vi "ctet_mux_User Main.vi"() -> ()   [LabVIEW 2019, in "ctet_mux_User Library.lvlib"]
uses:
  ctet_mux_User Library.lvlib
  Servers/ctet_mux/ctet_mux Class/typeDefs/Server State Data.ctl
  Types/ctet_mux.ctl
  Servers/ctet_mux/ctet_mux Class/ctet_mux.lvclass/ctet_mux.ctl
  Servers/ctet_mux/ctet_mux Class/ctet_mux.lvclass
panel:
  in  "Stop":bool
  in  "Server Address":string="0.0.0.0:50051"
  in  "Server Certificate File (.crt)":path
  in  "Server Key File (.key)":path
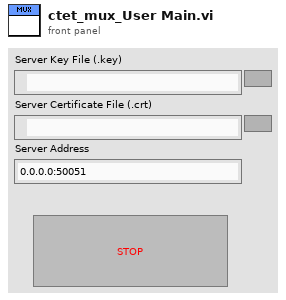
[diagram p1: front panel]
types:
  T1 = typedef "ctet_mux_User Library.lvlib/ctet_mux.ctl" = cluster{"MUXSession":refnum<k15>}
  T2 = typedef "ctet_mux.lvlib/ctet_mux.lvclass/Server State Data.ctl" = cluster{"Data":string}
  T3 = typedef "ctet_mux.lvlib/ctet_mux.lvclass/Server gRPC UEs.ctl" = cluster{"Invoke gRPC UE":refnum<user-event>, "Query gRPC UE":refnum<user-event>, "Register gRPC UE":refnum<user-event>, "OpenMUXSession gRPC UE":refnum<user-event>, "CloseMUXSession gRPC UE":refnum<user-event>, "OpenMUXChannel gRPC UE":refnum<user-event>, "CloseMUXChannel gRPC UE":refnum<user-event>, "OpenMUXRelay gRPC UE":refnum<user-event>, "CloseMUXRelay gRPC UE":refnum<user-event>, "CloseMUXAllRelays gRPC UE":refnum<user-event>, "DisconnectAllMUXChannels gRPC UE":refnum<user-event>, "ResetMUX gRPC UE":refnum<user-event>, "GetMUXStatus gRPC UE":refnum<user-event>, "GetMUXChannelNames gRPC UE":refnum<user-event>, "GetMUXRelayInfo gRPC UE":refnum<user-event>}
  T4 = typedef "ctet_mux.lvlib/gprc-lvsupport.lvlib/grpcId.ctl" = u64
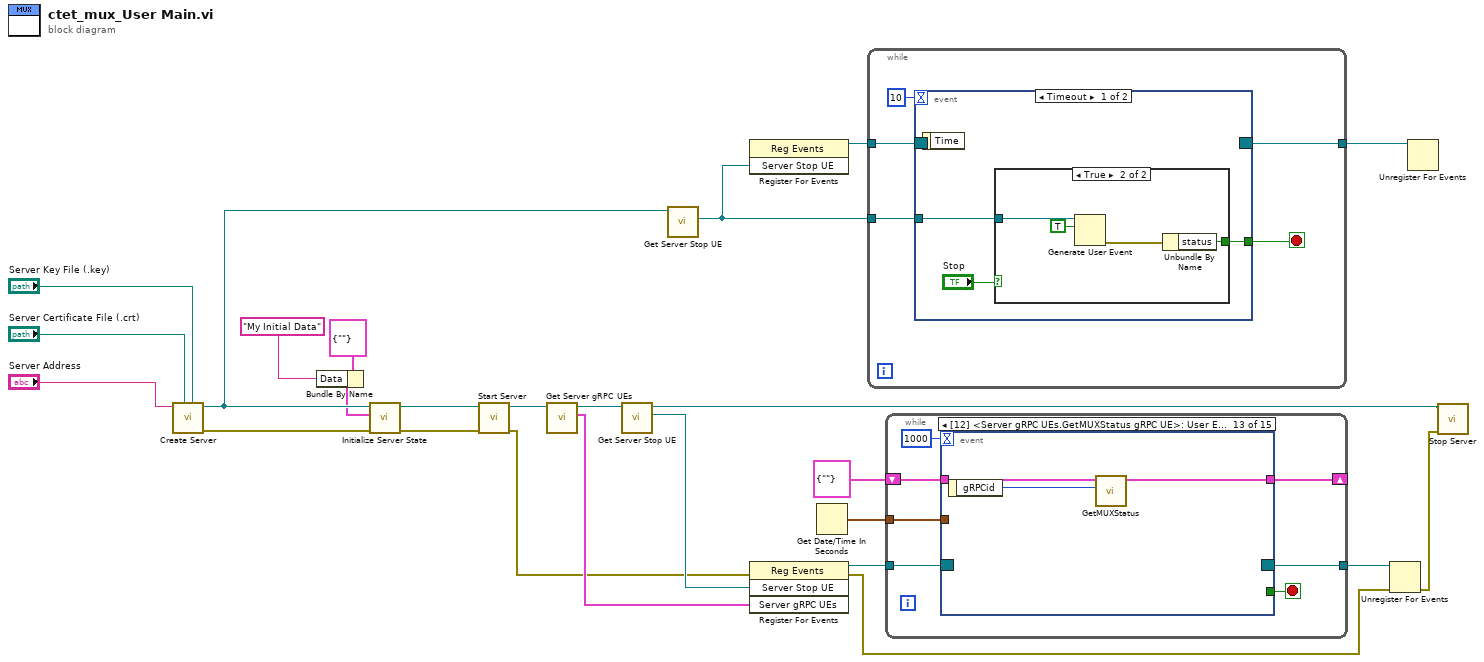
[diagram p0: block diagram]
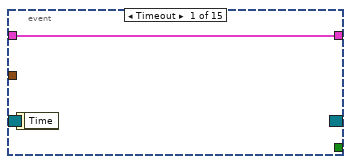
[diagram p2: hidden frame]
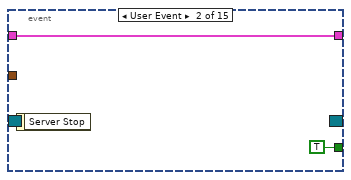
[diagram p3: hidden frame]
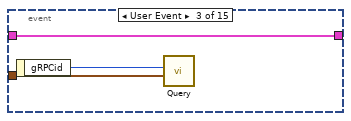
[diagram p4: hidden frame]
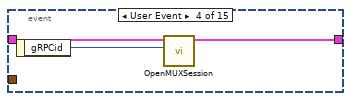
[diagram p5: hidden frame]
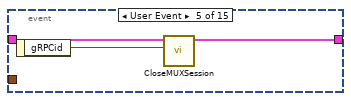
[diagram p6: hidden frame]
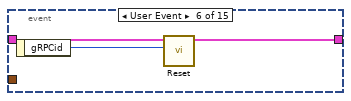
[diagram p7: hidden frame]
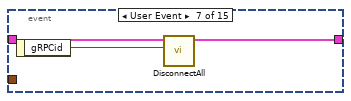
[diagram p8: hidden frame]
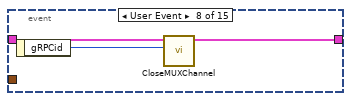
[diagram p9: hidden frame]
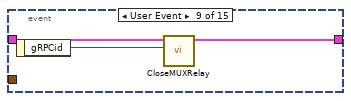
[diagram p10: hidden frame]
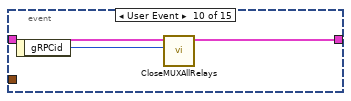
[diagram p11: hidden frame]
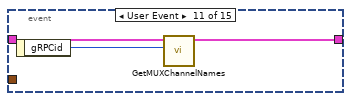
[diagram p12: hidden frame]
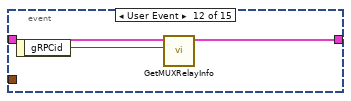
[diagram p13: hidden frame]
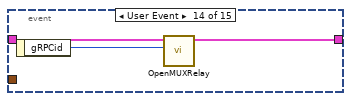
[diagram p14: hidden frame]
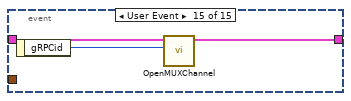
[diagram p15: hidden frame]
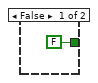
[diagram p16: hidden frame]
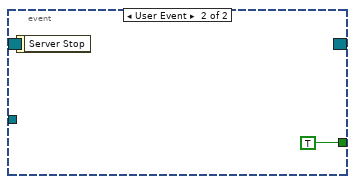
[diagram p17: hidden frame]
diagram:
  n1 = call "Create Server.vi"("Server Key File (.key)"="Server Key File (.key)", "Server Certificate File (.crt)"="Server Certificate File (.crt)", "Server Address"="Server Address") -> ("error out"=w19:errorcluster, "gRPC Server out"=w16:refnum<class "ctet_mux.lvclass">)  [unwired: 7 in]
  n2 = Bundle By Name(cluster=T2 {"Data"=""} ("Initial State"), "Data"="My Initial Data") -> (w14:T2)
  n3 = call "Initialize Server State.vi"("error in (no error)"=w19, "Initial State"=w14, "gRPC Server in"=w16) -> ("error out"=w18:errorcluster, "gRPC Server out"=w17:refnum<class "ctet_mux.lvclass">)  [unwired: 7 in]
  n4 = call "Start Server.vi"("error in (no error)"=w18, "gRPC Server in"=w17) -> ("error out"=w6:errorcluster, "gRPC Server out"=w7:refnum<class "ctet_mux.lvclass">)  [unwired: 8 in]
  n5 = call "Get Server gRPC UEs.vi"("OOP Server in"=w7) -> ("Server gRPC UEs"=w10:T3, "OOP Server out"=w12:refnum<class "ctet_mux.lvclass">)  [unwired: 9 in]
  n6 = call "Get Server Stop UE.vi"("OOP Server in"=w12) -> ("Server Stop UE"=w11:refnum<user-event>, "OOP Server out"=w4:refnum<class "ctet_mux.lvclass">)  [unwired: 9 in]
  n7 = call "Get Server Stop UE.vi"("OOP Server in"=w16) -> ("Server Stop UE"=w20:refnum<user-event>)  [unwired: 9 in, 1 out]
  n8 = register-events(w20) -> (reference out=w22:refnum<event-registration>)  [unwired: 2 in, 1 out]
  n9 = register-events(error in=w6, w11, w10) -> (reference out=w9:refnum<event-registration>, error out=w5:errorcluster)  [unwired: 1 in]
  n10 = Get Date/Time In Seconds() -> (seconds since 1Jan1904=w2:timestamp)
  n11 = while {
    tunnel: w20 -> [w30]
    tunnel: w22 -> [w29]
    tunnel: [w27] -> w21
    stop <- w28 stop-if-true
    n12 = event shown="[0] Timeout" {
      selector: w29 -> [_ _]
      dyn-events: [_ _] -> w27
      timeout: 10 -> [_ _]
      tunnel: w30 -> [w33 _]
      tunnel: [w32 TRUE] -> w28
      event Timeout {
        n13 = event-data() -> ()  [unwired: 1 in, 1 out]
        n14 = case shown="True" "Stop" {
          tunnel: w33 -> [_ w36]
          tunnel: [FALSE ("status") w35] -> w32
          frame False {
          }
          frame True {
            n15 = Generate User Event(user event=w36, event data cluster=TRUE ("event data")) -> (error out=w37:errorcluster)  [unwired: 2 in, 1 out]
            n16 = Unbundle By Name(w37) -> ("status"=w35:bool)
          }
        }
      }
      event User Event {
        n17 = event-data() -> ()  [unwired: 1 in, 1 out]
      }
    }
  }
  n18 = while {
    tunnel: w9 -> [w46]
    tunnel: [w44] -> w8
    tunnel: w2 -> [w42]
    shift-right: [w40] -> _
    shift-left: T1 {"MUXSession"=""} ("ctet_mux in") -> [w41]
    stop <- w45 stop-if-true
    n19 = event "RPC Methods Event Structure" shown="[12] <Server gRPC UEs.GetMUXStatus gRPC UE>: User Event" {
      selector: w46 -> [_ _ _ _ _ _ _ _ _ _ _ _ _ _ _]
      dyn-events: [_ _ _ _ _ _ _ _ _ _ _ _ _ _ _] -> w44
      timeout: 1000 -> [_ _ _ _ _ _ _ _ _ _ _ _ _ _ _]
      tunnel: [_ TRUE _ _ _ _ _ _ _ _ _ _ _ _ _] -> w45
      tunnel: w42 -> [_ _ w51 _ _ _ _ _ _ _ _ _ _ _ _]
      tunnel: w41 -> [w47 w48 w50 w54 w57 w60 w63 w66 w69 w72 w75 w78 w81 w84 w87]
      tunnel: [w47 w48 w50 w53 w56 w59 w62 w65 w68 w71 w74 w77 w80 w83 w86] -> w40
      event Timeout {
        n20 = event-data() -> ()  [unwired: 1 in, 1 out]
      }
      event User Event {
        n21 = event-data() -> ()  [unwired: 1 in, 1 out]
      }
      event User Event {
        n22 = event-data() -> ("gRPCid"=w52:T4)  [unwired: 1 in]
        n23 = call "Query.vi"("current time"=w51, "gRPCid"=w52) -> ()  [unwired: 9 in, 1 out]
      }
      event User Event {
        n24 = event-data() -> ("gRPCid"=w55:T4)  [unwired: 1 in]
        n25 = call "OpenMUXSession.vi"("gRPCid"=w55, "ctet_mux in"=w54) -> ("ctet_mux out"=w53:T1)  [unwired: 8 in, 1 out]
      }
      event User Event {
        n26 = event-data() -> ("gRPCid"=w58:T4)  [unwired: 1 in]
        n27 = call "CloseMUXSession.vi"("gRPCid"=w58, "ctet_mux in"=w57) -> ("ctet_mux out"=w56:T1)  [unwired: 8 in, 1 out]
      }
      event User Event {
        n28 = event-data() -> ("gRPCid"=w61:T4)  [unwired: 1 in]
        n29 = call "Reset.vi"("gRPCid"=w61, "ctet_mux in"=w60) -> ("ctet_mux out"=w59:T1)  [unwired: 8 in, 1 out]
      }
      event User Event {
        n30 = event-data() -> ("gRPCid"=w64:T4)  [unwired: 1 in]
        n31 = call "DisconnectAll.vi"("gRPCid"=w64, "ctet_mux in"=w63) -> ("ctet_mux out"=w62:T1)  [unwired: 8 in, 1 out]
      }
      event User Event {
        n32 = event-data() -> ("gRPCid"=w67:T4)  [unwired: 1 in]
        n33 = call "CloseMUXChannel.vi"("gRPCid"=w67, "ctet_mux in"=w66) -> ("ctet_mux out"=w65:T1)  [unwired: 8 in, 1 out]
      }
      event User Event {
        n34 = event-data() -> ("gRPCid"=w70:T4)  [unwired: 1 in]
        n35 = call "CloseMUXRelay.vi"("gRPCid"=w70, "ctet_mux in"=w69) -> ("ctet_mux out"=w68:T1)  [unwired: 8 in, 1 out]
      }
      event User Event {
        n36 = event-data() -> ("gRPCid"=w73:T4)  [unwired: 1 in]
        n37 = call "CloseMUXAllRelays.vi"("gRPCid"=w73, "ctet_mux in"=w72) -> ("ctet_mux out"=w71:T1)  [unwired: 8 in, 1 out]
      }
      event User Event {
        n38 = event-data() -> ("gRPCid"=w76:T4)  [unwired: 1 in]
        n39 = call "GetMUXChannelNames.vi"("gRPCid"=w76, "ctet_mux in"=w75) -> ("ctet_mux out"=w74:T1)  [unwired: 8 in, 1 out]
      }
      event User Event {
        n40 = event-data() -> ("gRPCid"=w79:T4)  [unwired: 1 in]
        n41 = call "GetMUXRelayInfo.vi"("gRPCid"=w79, "ctet_mux in"=w78) -> ("ctet_mux out"=w77:T1)  [unwired: 8 in, 1 out]
      }
      event User Event {
        n42 = event-data() -> ("gRPCid"=w82:T4)  [unwired: 1 in]
        n43 = call "GetMUXStatus.vi"("gRPCid"=w82, "ctet_mux in"=w81) -> ("ctet_mux out"=w80:T1)  [unwired: 8 in, 1 out]
      }
      event User Event {
        n44 = event-data() -> ("gRPCid"=w85:T4)  [unwired: 1 in]
        n45 = call "OpenMUXRelay.vi"("gRPCid"=w85, "ctet_mux in"=w84) -> ("ctet_mux out"=w83:T1)  [unwired: 8 in, 1 out]
      }
      event User Event {
        n46 = event-data() -> ("gRPCid"=w88:T4)  [unwired: 1 in]
        n47 = call "OpenMUXChannel.vi"("gRPCid"=w88, "ctet_mux in"=w87) -> ("ctet_mux out"=w86:T1)  [unwired: 8 in, 1 out]
      }
    }
  }
  n48 = Unregister For Events(event registration refnum=w8, error in=w5) -> (error out=w3:errorcluster)
  n49 = Unregister For Events(event registration refnum=w21) -> ()  [unwired: 1 in, 1 out]
  n50 = call "Stop Server.vi"("error in (no error)"=w3, "gRPC Server in"=w4) -> ()  [unwired: 9 in, 1 out]
